vi "Choose Selected Control.vi"(11 "reference":refnum<vi>) -> (3 "appended array":refnum<vi>[](array[refnum]), 5 "Position":T1, 7 "Owner":refnum<vi>)   [LabVIEW 2015]
uses:
  <vilib>/Utility/miscctls.llb/LVPositionTypeDef.ctl
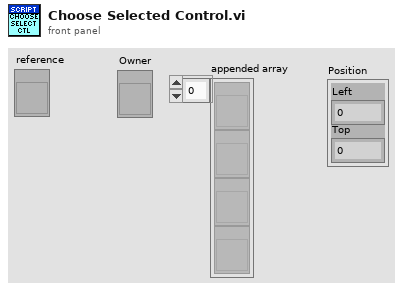
[diagram p1: front panel]
types:
  T1 = typedef "LVPositionTypeDef.ctl" = cluster{"Left":i32, "Top":i32}
  T2 = typedef "LVRectTypeDef.ctl" = cluster{"Left":i16, "Top":i16, "Right":i16, "Bottom":i16}
  T3 = typedef "LVPointTypeDef.ctl" = cluster{"Horizontal":i16, "Vertical":i16}
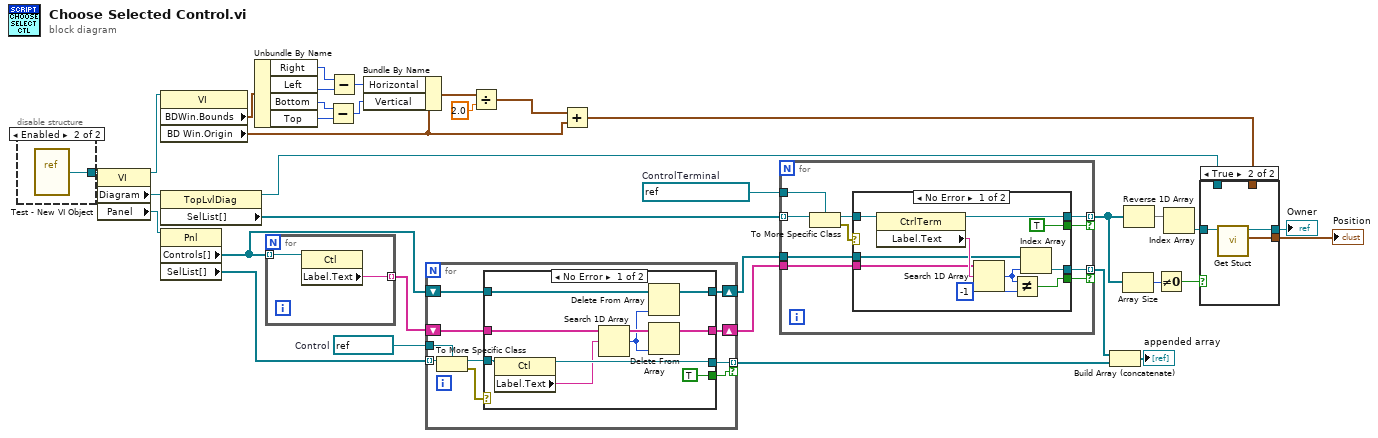
[diagram p0: block diagram]
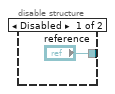
[diagram p2: hidden frame]
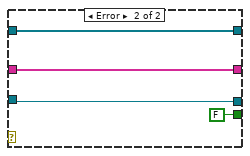
[diagram p4: hidden frame]
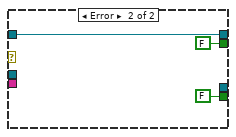
[diagram p5: hidden frame]
diagram:
  w28 = refnum<vi> refnum  # ControlTerminal
  w30 = refnum<vi> refnum  # Control
  n1 = disable-structure shown="Enabled" {
    disable-tunnel: ["reference" w37] -> w22
    frame Disabled {
    }
    frame Enabled {
      n2 = vi-ref "Test - New VI Object.vi"() -> (w37:refnum<vi>)
    }
  }
  n3 = property class="VI"(reference=w22) -> (reference out=w6:refnum<vi>, "Diagram"=w35:refnum<vi>, "Panel"=w34:refnum<vi>)  [unwired: 1 in, 1 out]
  n4 = property class="VI"(reference=w6) -> ("BDWin.Bounds"=w9:T2, "BD Win.Origin"=w2:T3)  [unwired: 1 in, 2 out]
  n5 = property class="TopLvlDiag"(reference=w35) -> (reference out=w5:refnum<vi>, "SelList[]"=w33:refnum<vi>[])  [unwired: 1 in, 1 out]
  n6 = property class="Pnl"(reference=w34) -> ("Controls[]"=w27:refnum<vi>[], "SelList[]"=w32:refnum<vi>[])  [unwired: 1 in, 2 out]
  n7 = Unbundle By Name(w9) -> ("Right"=w10:i16, "Left"=w11:i16, "Bottom"=w8:i16, "Top"=w14:i16)
  n8 = for {
    tunnel: w27 -> [w39] mode=indexing
    tunnel: [w38] -> w31 mode=indexing
    n9 = property class="Ctl"(reference=w39) -> ("Label.Text"=w38:string)  [unwired: 1 in, 2 out]
  }
  n10 = Subtract(x=w8, y=w14) -> (x-y=w13:i16)
  n11 = Subtract(x=w10, y=w11) -> (x-y=w12:i16)
  n12 = Bundle By Name(cluster=w2, "Horizontal"=w12, "Vertical"=w13) -> (w15:T3)
  n13 = for {
    tunnel: w32 -> [w49] mode=indexing
    tunnel: [w47] -> w24 mode=indexing if=w44
    tunnel: w30 -> [w46]
    shift-right: [w42] -> w29
    shift-left: w31 -> [w43]
    shift-right: [w40] -> w26
    shift-left: w27 -> [w41]
    n14 = To More Specific Class(target class=w46, reference=w49) -> (specific class reference=w48:refnum<vi>, error out=w45:errorcluster)  [unwired: 1 in]
    n15 = case shown="No Error" w45 {
      tunnel: w48 -> [w58 w61]
      tunnel: [w57 w61] -> w47
      tunnel: [TRUE FALSE] -> w44
      tunnel: w43 -> [w54 w60]
      tunnel: [w53 w60] -> w42
      tunnel: w41 -> [w52 w59]
      tunnel: [w50 w59] -> w40
      frame No Error {
        n16 = property class="Ctl"(reference=w58) -> (reference out=w57:refnum<vi>, "Label.Text"=w55:string)  [unwired: 1 in, 1 out]
        n17 = Search 1D Array(1D array=w54, element=w55) -> (index of element=w51:i32)  [unwired: 1 in]
        n18 = Delete From Array(array=w52, index=w51) -> (array with subset deleted=w50:refnum<vi>[])  [unwired: 1 in, 1 out]
        n19 = Delete From Array(array=w54, index=w51) -> (array with subset deleted=w53:string[])  [unwired: 1 in, 1 out]
      }
      frame Error {
      }
    }
  }
  n20 = Divide(x=w15, y=2.0) -> (x/y=w16:cluster{"Horizontal":dbl, "Vertical":dbl})
  n21 = Add(x=w16, y=w2) -> (x+y=w7:cluster{"Horizontal":dbl, "Vertical":dbl})
  n22 = for {
    tunnel: w33 -> [w72] mode=indexing
    tunnel: w28 -> [w68]
    tunnel: w26 -> [w67]
    tunnel: w29 -> [w69]
    tunnel: [w66] -> w25 mode=indexing if=w65
    tunnel: [w64] -> w1 mode=indexing if=w63
    n23 = To More Specific Class(target class=w68, reference=w72) -> (specific class reference=w70:refnum<vi>, error out=w71:errorcluster)  [unwired: 1 in]
    n24 = case shown="No Error" w71 {
      tunnel: w70 -> [w82 w84]
      tunnel: w69 -> [w80 _]
      tunnel: w67 -> [w79 _]
      tunnel: [w78 _] -> w66
      tunnel: [w75 FALSE] -> w65
      tunnel: [w74 w84] -> w64
      tunnel: [TRUE FALSE] -> w63
      frame No Error {
        n25 = property class="CtrlTerm"(reference=w82) -> (reference out=w74:refnum<vi>, "Label.Text"=w81:string)  [unwired: 1 in, 1 out]
        n26 = Search 1D Array(1D array=w80, element=w81) -> (index of element=w77:i32)  [unwired: 1 in]
        n27 = Not Equal?(x=w77, y=-1) -> (x != y?=w75:bool)
        n28 = Index Array(array=w79, index=w77) -> (element=w78:refnum<vi>)
      }
      frame Error {
      }
    }
  }
  n29 = Build Array (concatenate)(w25, w24) -> (→"appended array":refnum<vi>[])
  n30 = Array Size(array=w1) -> (size(s)=w19:i32)
  n31 = Reverse 1D Array(array=w1) -> (reversed array=w21:refnum<vi>[])
  n32 = Not Equal To 0?(x=w19) -> (x != 0?=w18:bool)
  n33 = Index Array(array=w21) -> (element=w20:refnum<vi>)  [unwired: 1 in]
  n34 = case shown="True" w18 {
    tunnel: w20 -> [_ w90]
    tunnel: [w86 w88] -> w3
    tunnel: w7 -> [w87 _]
    tunnel: [w87 w89] -> w4
    tunnel: w5 -> [w86 _]
    frame False {
    }
    frame True {
      n35 = call "Get Stuct.vi"("reference"=w90) -> ("Position"=w89:T1, "ower reference"=w88:refnum<vi>)  [unwired: 9 in]
    }
  }
  "Position" <- w4
  "Owner" <- w3
